vi "LV2GOrderList.vi"(7 "Operation":T1, 8 "error in (no error)":errorcluster, 11 "Orders":string[][](array[string])) -> (0 "error out":errorcluster, 3 "Orders out":string[][](array[string]))   [LabVIEW 2011]
uses:
  Strict Type Controls/Settings Operation.ctl
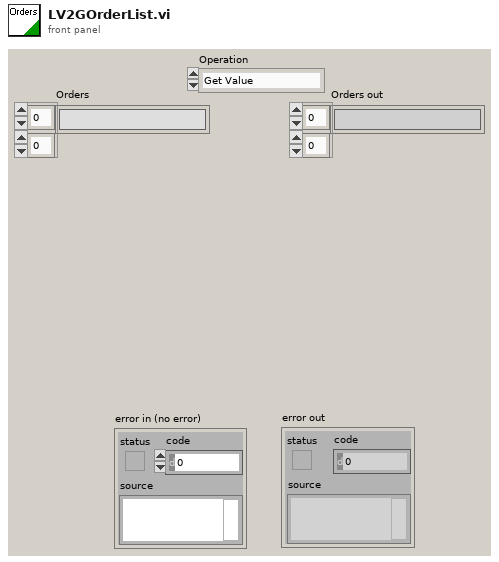
[diagram p1: front panel]
types:
  T1 = typedef "Settings Operation.ctl" = enum8{"Get Value", "Set Value", "Read File", "Write File", "Write Stored Value"}
  T2 = enum16{"open", "replace", "create", "open or create", "replace or create", "replace or create with confirmation"}
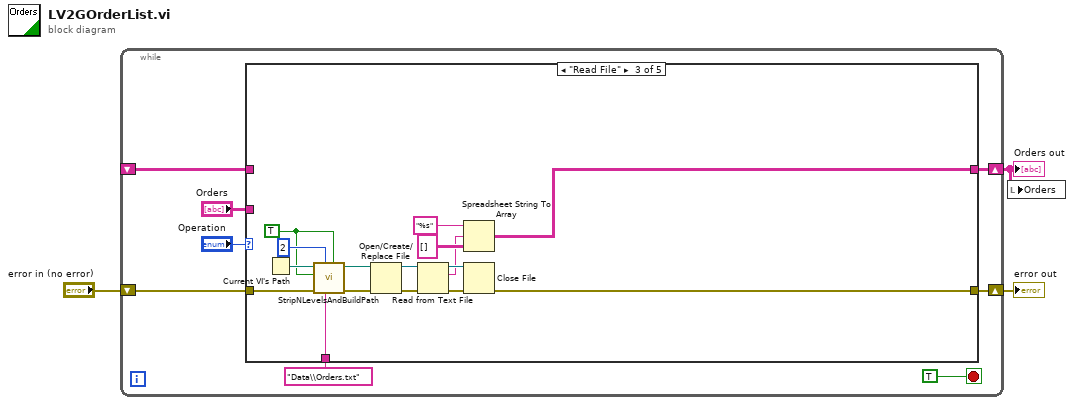
[diagram p0: block diagram]
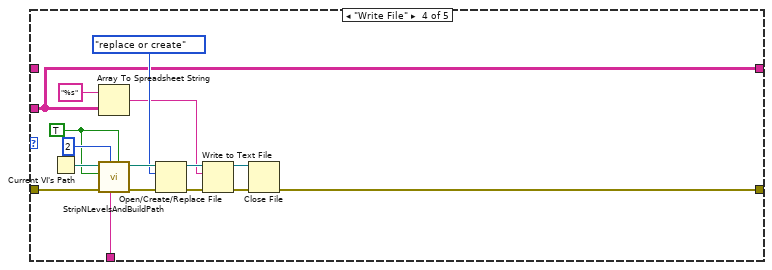
[diagram p4: hidden frame]
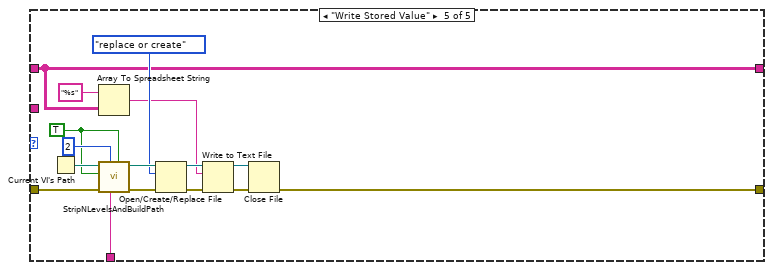
[diagram p5: hidden frame]
diagram:
  n1 = while {
    shift-right: [w10] -> w2
    shift-left: _ -> [w11]
    shift-right: [w7] -> w1
    shift-left: "error in (no error)" -> [w8]
    stop <- TRUE stop-if-true
    n2 = case shown="\"Read File\"" "Operation" {
      tunnel: w11 -> [w13 _ _ _ w48]
      tunnel: [w13 w15 w18 w34 w48] -> w10
      tunnel: "Orders" -> [_ w15 _ w34 _]
      tunnel: w8 -> [w12 w14 w28 w46 w62]
      tunnel: [w12 w14 w20 w37 w53] -> w7
      tunnel: "Data\\Orders.txt" ("Build Path") -> [_ _ w27 w36 w52]
      frame "Get Value" {
      }
      frame "Set Value" {
      }
      frame "Read File" {
        w29 = TRUE ("Is File?")
        n3 = Current VI's Path() -> (path=w31:path)
        n4 = call "StripNLevelsAndBuildPath.vi"("Create Folders"=w29, "Build Path"=w27, "Strip Levels"=2, "error in(no error)"=w28, "Is File"=w29, "Path In"=w31) -> ("error out"=w21:errorcluster, "Path Out"=w22:path)  [unwired: 4 out]
        n5 = Open/Create/Replace File(file path (use dialog)=w22, error in=w21) -> (refnum out=w26:refnum<file>, error out=w25:errorcluster)  [unwired: 5 out]
        n6 = Read from Text File(file (use dialog)=w26, error in=w25) -> (refnum out=w23:refnum<file>, text=w17:string, error out=w24:errorcluster)  [unwired: 3 out]
        n7 = Spreadsheet String To Array(format string="%s", spreadsheet string=w17, array type (2D Dbl)=string[][] []) -> (array=w18:string[][])  [unwired: 1 out]
        n8 = Close File(refnum=w23, error in=w24) -> (error out=w20:errorcluster)  [unwired: 1 out]
      }
      frame "Write File" {
        w44 = TRUE ("Is File?")
        n9 = Current VI's Path() -> (path=w47:path)
        n10 = Array To Spreadsheet String(array=w34, 3:"%s" ("format string")) -> (spreadsheet string=w32:string)  [unwired: 1 out]
        n11 = call "StripNLevelsAndBuildPath.vi"("Create Folders"=w44, "Build Path"=w36, "Strip Levels"=2, "error in(no error)"=w46, "Is File"=w44, "Path In"=w47) -> ("error out"=w38:errorcluster, "Path Out"=w43:path)  [unwired: 4 out]
        n12 = Open/Create/Replace File(file path (use dialog)=w43, error in=w38, operation (0:open)=T2."replace or create") -> (refnum out=w42:refnum<file>, error out=w41:errorcluster)  [unwired: 4 out]
        n13 = Write to Text File(file (use dialog)=w42, text=w32, error in=w41) -> (refnum out=w39:refnum<file>, error out=w40:errorcluster)  [unwired: 2 out]
        n14 = Close File(refnum=w39, error in=w40) -> (error out=w37:errorcluster)  [unwired: 1 out]
      }
      frame "Write Stored Value" {
        w60 = TRUE ("Is File?")
        n15 = Current VI's Path() -> (path=w63:path)
        n16 = Array To Spreadsheet String(array=w48, 3:"%s" ("format string")) -> (spreadsheet string=w49:string)  [unwired: 1 out]
        n17 = call "StripNLevelsAndBuildPath.vi"("Create Folders"=w60, "Build Path"=w52, "Strip Levels"=2, "error in(no error)"=w62, "Is File"=w60, "Path In"=w63) -> ("error out"=w54:errorcluster, "Path Out"=w59:path)  [unwired: 4 out]
        n18 = Open/Create/Replace File(file path (use dialog)=w59, error in=w54, operation (0:open)=T2."replace or create") -> (refnum out=w58:refnum<file>, error out=w57:errorcluster)  [unwired: 4 out]
        n19 = Write to Text File(file (use dialog)=w58, text=w49, error in=w57) -> (refnum out=w55:refnum<file>, error out=w56:errorcluster)  [unwired: 2 out]
        n20 = Close File(refnum=w55, error in=w56) -> (error out=w53:errorcluster)  [unwired: 1 out]
      }
    }
  }
  "error out" <- w1
  "Orders out" <- w2
  n21 = local write "Orders"(w2) -> ()
